vi "Reset Analyzer.vi"(0 "VISA Session In":refnum<visa-resource-name>="OXYMAT", 1 "Target Address":u8=16 format="%.0x", 2 "Source Address":u8=208 format="%.0x", 11 "error in (no error)":errorcluster) -> (4 "VISA Session Out":refnum<visa-resource-name>, 6 "Message Header":T1 {"Source Address" format="%.0x"; "Target Address" format="%.0x"}, 13 "Success":bool, 15 "error out":errorcluster)   [LabVIEW 2020, in "Siemens ELAN.lvlib"]
doc: "Using the Siemens ELAN protocol, resets the addressed analyzer. Returns a boolean indicating that the addressed device provided a valid response.\n\n$Revision:: 0 $\n$Modtime:: yy-mm-dd hh:mm $\n$Author:: Dboyd $"
uses:
  Siemens ELAN.lvlib
  Message Header.ctl
  Channel Status.ctl
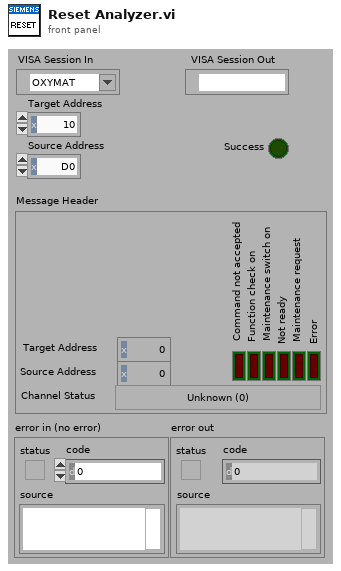
[diagram p1: front panel]
types:
  T1 = typedef "Siemens ELAN.lvlib/Message Header.ctl" = cluster{"Target Address":u8, "Source Address":u8, "Error":bool, "Maintenance request":bool, "Not ready":bool, "Maintenance switch on":bool, "Function check on":bool, "Command not accepted":bool, "Channel Status":T2}
  T2 = typedef "Siemens ELAN.lvlib/Channel Status.ctl" = enum8{"Unknown (0)", "Warm-up", "Pause", "Standby", "Measure", "Zero calibration", "Adjust component slope", "Unknown (7)", "Adjust curve dip", "Adjust linearization sensitivity", "Adjust temperature compensation", "Adjust pressure compensation", "Adjust linearization zero", "Adjust flow sensor", "Autocal", "Adjust phase", "Zero calibration of O2 sensor", "Synchronous zero calibration", "Purging for synchronous zero calibration", "Adjust analog output", "Adjust analog input", "Cleaning", "Unknown (>21)"}
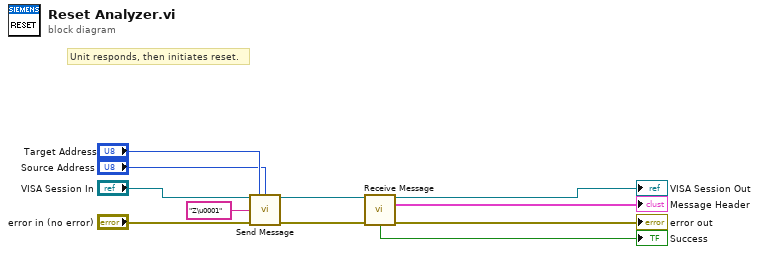
[diagram p0: block diagram]
diagram:
  # "Unit responds, then initiates reset."
  n1 = call "Send Message.vi"("VISA Session In"="VISA Session In", "Target Address"="Target Address", "Source Address"="Source Address", "Command"="Z\u0001", "error in (no error)"="error in (no error)") -> ("VISA Session Out"=w11:refnum<visa-resource-name>, "error out"=w10:errorcluster)  [unwired: 8 in, 1 out]
  n2 = call "Receive Message.vi"("VISA Session In"=w11, "error in (no error)"=w10) -> ("VISA Session Out"=→"VISA Session Out":refnum<visa-resource-name>, "Message Header"=→"Message Header":T1, "Success"=→"Success":bool, "error out"=→"error out":errorcluster)  [unwired: 8 in, 2 out]
